vi "HISTO_CLEAN.vi"(0 "TCP Network Connection in":refnum<k5>, 5 "error in (no error)":errorcluster) -> (14 "TCP Network Connection out":refnum<k5>, 15 "DEC_STATUS":u8[](array[numeric]), 19 "error out":errorcluster)   [LabVIEW 2019, in "Histogram.lvlib"]
uses:
  Histogram.lvlib
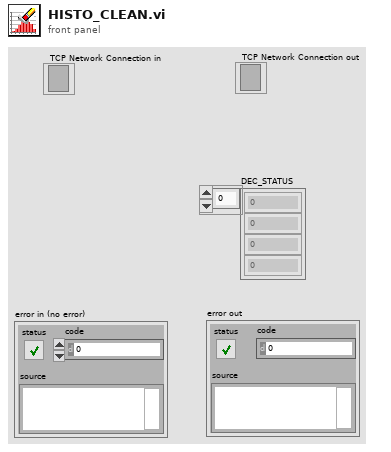
[diagram p1: front panel]
types:
  T1 = enum16{"big-endian, network order", "native, host order", "little-endian"}
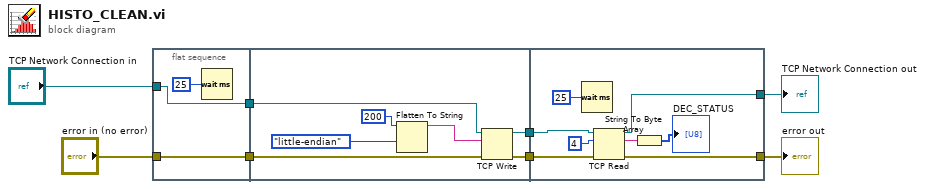
[diagram p0: block diagram]
diagram:
  n1 = flat-sequence {
    tunnel: [w10] -> w4
    tunnel: [w11] -> w3
    tunnel: "error in (no error)" -> [w11]
    tunnel: "TCP Network Connection in" -> [w10]
    tunnel: w4 -> [w18]
    tunnel: w3 -> [w17]
    tunnel: [w16] -> w2
    tunnel: [w15] -> w1
    tunnel: [w23] -> w6
    tunnel: [w24] -> w5
    tunnel: w2 -> [w26]
    tunnel: w1 -> [w25]
    frame #0 {
      n2 = Wait (ms)(milliseconds to wait=u32 25) -> ()  [unwired: 1 out]
    }
    frame #1 {
      n3 = Flatten To String(anything=u32 200 ("element"), byte order (0:big-endian, network order)=T1."little-endian") -> (data string=w12:string)  [unwired: 2 in, 2 out]
      n4 = TCP Write(connection ID=w18, data in=w12, error in (no error)=w17) -> (connection ID out=w16:refnum<k5>, error out=w15:errorcluster)  [unwired: 1 in, 1 out]
    }
    frame #2 {
      n5 = Wait (ms)(milliseconds to wait=u32 25) -> ()  [unwired: 1 out]
      n6 = TCP Read(connection ID=w26, bytes to read=4, error in (no error)=w25) -> (connection ID out=w24:refnum<k5>, data out=w20:string, error out=w23:errorcluster)  [unwired: 2 in]
      n7 = String To Byte Array(string=w20) -> (unsigned byte array=→"DEC_STATUS":u8[])
    }
  }
  "error out" <- w6
  "TCP Network Connection out" <- w5
